vi "Start.vi"(0 "reference in":refnum<class "ConveyorBelt.lvclass">, 5 "error in (no error)":errorcluster) -> (14 "reference out":refnum<class "ConveyorBelt.lvclass">, 19 "error out":errorcluster)   [LabVIEW 2014, in "ConveyorBelt.lvclass"]
uses:
  ConveyorBelt.lvclass
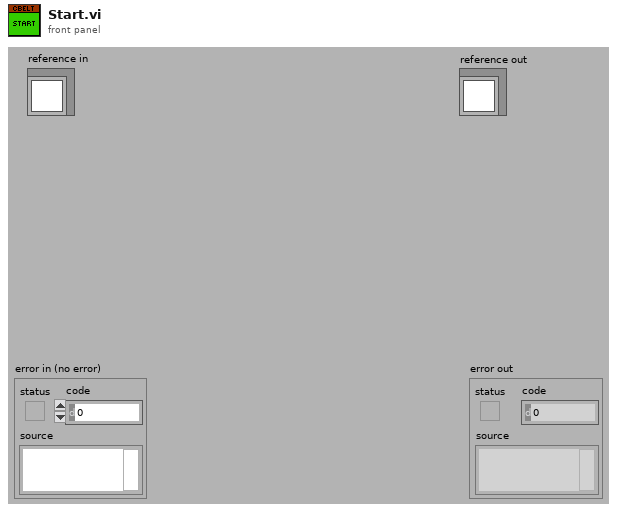
[diagram p1: front panel]
types:
  T1 = typedef "ConveyorBelt.lvclass/ObjectAttributes.ctl" = cluster{"Right":bool, "Running":bool, "ConveyorBeltRef":refnum<vi>}
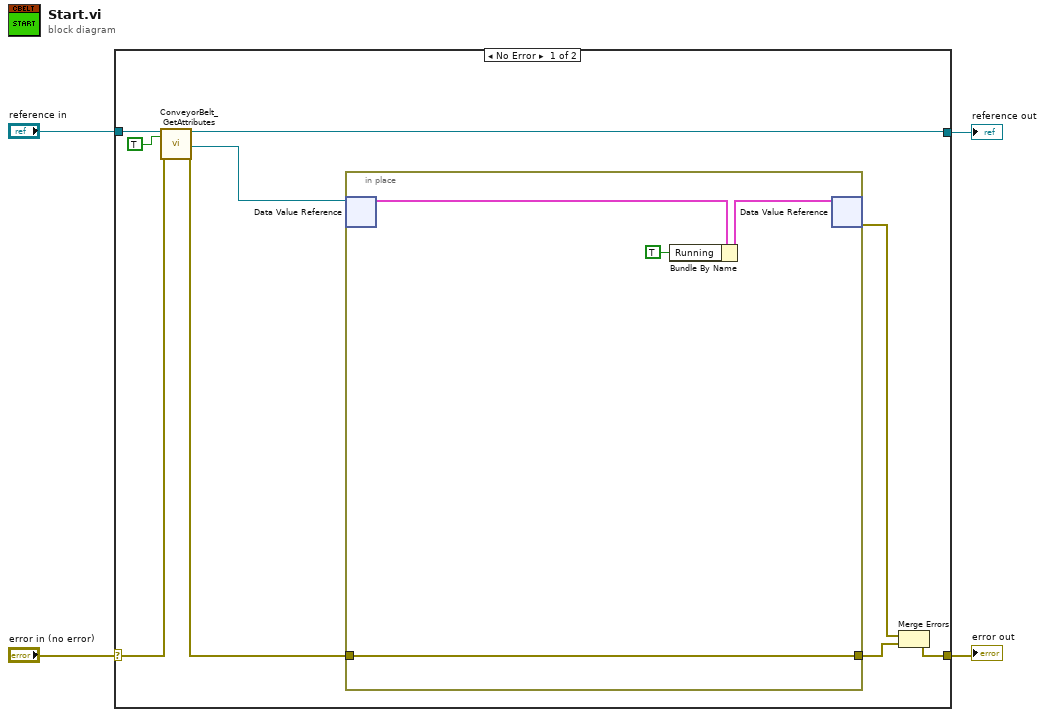
[diagram p0: block diagram]
diagram:
  n1 = case shown="No Error" "error in (no error)" {
    selector: "error in (no error)" -> [w10 w19]
    tunnel: [w12 w19] -> w3
    tunnel: [w8 w18] -> w1
    tunnel: "reference in" -> [w11 w18]
    frame No Error {
      n2 = call "ConveyorBelt_GetAttributes.vi"("reference in"=w11, "OnlyGetDvrReference(False)"=TRUE, "error in (no error)"=w10) -> ("reference out"=w8:refnum<class "ConveyorBelt.lvclass">, "DataRef"=w9:refnum<data-value>, "error out"=w6:errorcluster)  [unwired: 13 in, 1 out]
      n3 = in-place {
        in-place-border: w6 -> [w16]
        in-place-border: [w16] -> w5
        n4 = in-place-dvr #1(w9) -> (w15:T1)  [unwired: 1 out]
        n5 = Bundle By Name(cluster=w15, "Running"=TRUE) -> (w17:T1)
        n6 = in-place-dvr #1(w17) -> (w13:errorcluster)  [unwired: 1 out]
      }
      n7 = Merge Errors(w13, w5) -> (w12:errorcluster)
    }
    frame Error {
    }
  }
  "error out" <- w3
  "reference out" <- w1
